vi "HT3_Open.vi"(8 "error in":errorcluster, 11 "File Path":path) -> (0 "error out":errorcluster, 1 "Num Records":i64, 2 "Header":T2, 3 "refnum out":refnum<file>, 4 "Stop After (ms)":i32, 5 "Stop Reason":enum16{"timeover", "manual", "overflow"}(ring), 7 "Image Header":T1)   [LabVIEW 2009]
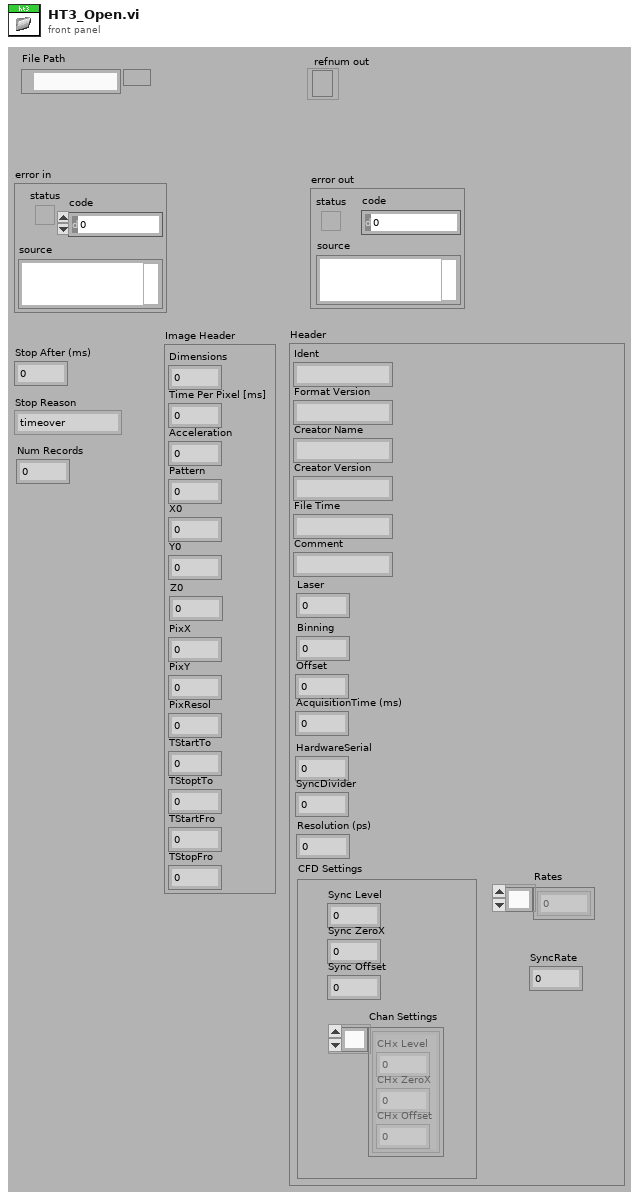
[diagram p1: front panel]
types:
  T1 = cluster{"Dimensions":i32, "Time Per Pixel [ms]":dbl, "Acceleration":i32, "Pattern":i32, "X0":sgl, "Y0":sgl, "Z0":dbl, "PixX":i32, "PixY":i32, "PixResol":sgl, "TStartTo":sgl, "TStoptTo":sgl, "TStartFro":sgl, "TStopFro":sgl}
  T2 = cluster{"Ident":string, "Format Version":string, "Creator Name":string, "Creator Version":string, "File Time":string, "Comment":string, "Laser":i32, "Binning":i32, "Offset":i32, "AcquisitionTime (ms)":i32, "HardwareSerial":i32, "SyncDivider":i32, "Resolution (ps)":dbl, "Rates":dbl[], "SyncRate":dbl, "CFD Settings":cluster{"Sync Level":i32, "Sync ZeroX":i32, "Sync Offset":i32, "Chan Settings":cluster{"CHx Level":i32, "CHx ZeroX":i32, "CHx Offset":i32}[]}}
  T3 = cluster{"Sync Level":i32, "Sync ZeroX":i32, "Sync Offset":i32, "Chan Settings":cluster{"CHx Level":i32, "CHx ZeroX":i32, "CHx Offset":i32}[]}
  T4 = cluster{"Ident":string, "Format Version":string, "Creator Name":string, "Creator Version":string, "File Time":string, "Comment":string, i32, "Binning":i32, "Offset":i32, "AcquisitionTime (ms)":i32, "HardwareSerial":i32, "SyncDivider":i32, "Resolution (ps)":dbl, i32[], "InpRate1":i32, "CFD Settings":cluster{"Sync Level":i32, "Sync ZeroX":i32, "Sync Offset":i32, "Chan Settings":cluster{"CHx Level":i32, "CHx ZeroX":i32, "CHx Offset":i32}[]}}
  T5 = enum16{"big-endian, network order", "native, host order", "little-endian"}
  T6 = enum16{"open", "replace", "create", "open or create", "replace or create", "replace or create with confirmation"}
  T7 = cluster{"Dimensions":i32, "Time Per Pixel [ms]":dbl, "Acceleration":i32, "Pattern":i32, "X0":sgl, "Y0":sgl, dbl, "PixX":i32, "PixY":i32, "PixResol":sgl, "TStartTo":sgl, "TStoptTo":sgl, "TStartFro":sgl, "TStopFro":sgl}
  T8 = cluster{"Strings[0]":string, "Strings[1]":string, "Strings[2]":string, "Strings[3]":string, "Strings[4]":string, "Strings[5]":string}
  T9 = cluster{"[0]":i32, "[1]":i32, "[2]":i32, "[3]":i32}
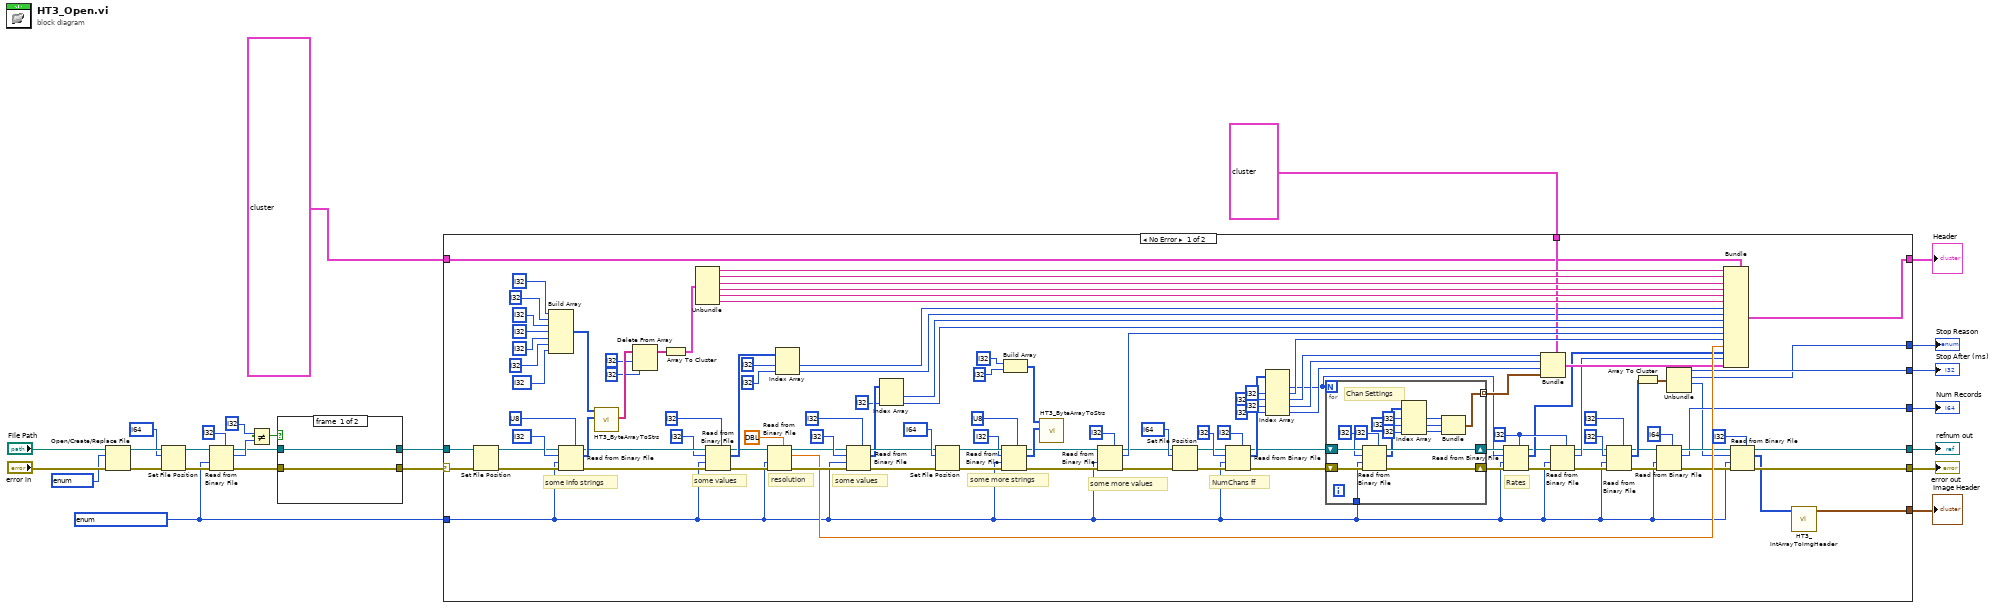
[diagram p0: block diagram]
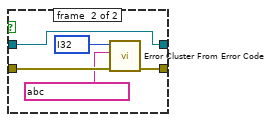
[diagram p2: hidden frame]
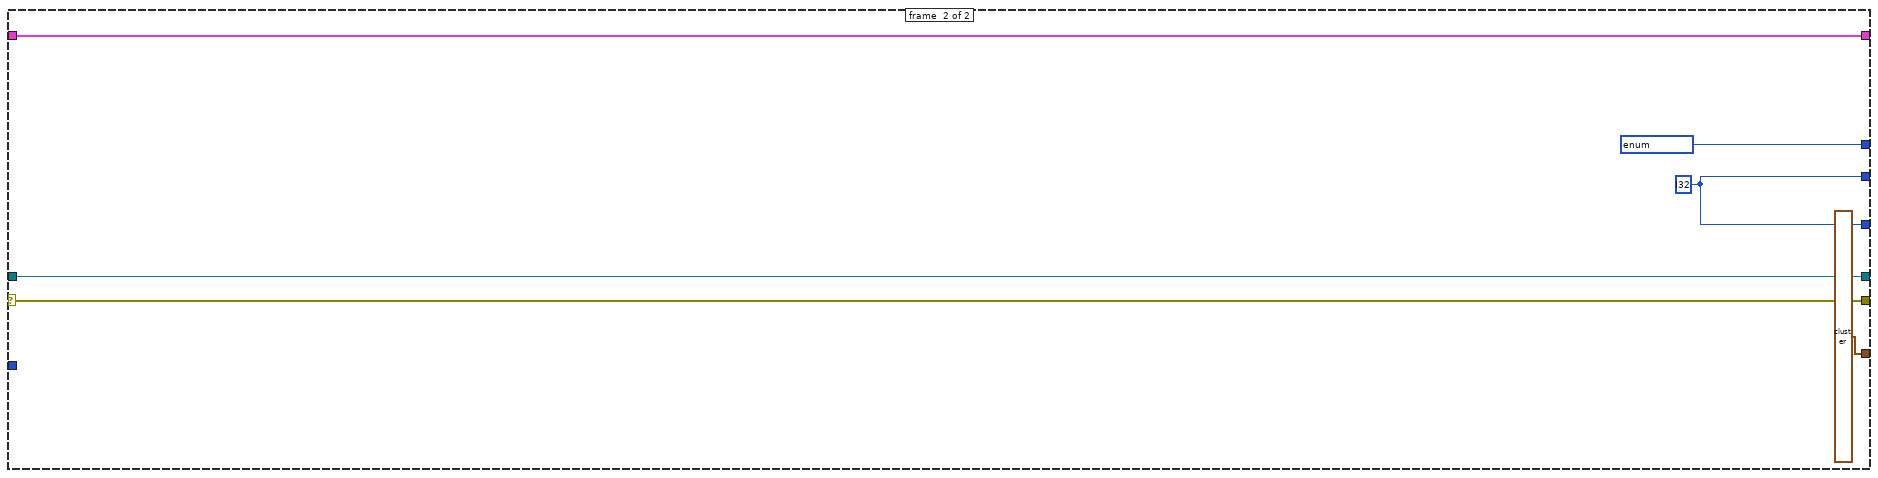
[diagram p3: hidden frame]
diagram:
  w12 = T5 ? ("byte order (0:big-endian, network order)")
  n1 = Open/Create/Replace File(file path (use dialog)="File Path", error in="error in", operation (0:open)=T6 ?) -> (refnum out=w15:refnum<file>, error out=w16:errorcluster)  [unwired: 4 out]
  n2 = Set File Position(offset (in bytes) (0)=i64 ?, refnum=w15, error in=w16) -> (refnum out=w11:refnum<file>, error out=w13:errorcluster)  [unwired: 1 out]
  n3 = Read from Binary File(5:i32 ?, 8:w13, 9:w12, 11:w11) -> (0:w6:errorcluster, 2:w9:i32, 3:w3:refnum<file>)  [unwired: 3 out]
  n4 = Not Equal?(x=i32 ?, y=w9) -> (x != y?=w7:bool)
  n5 = case shown="True" w7 {
    tunnel: w6 -> [w28 w33]
    tunnel: [w28 w32] -> w5
    tunnel: [w27 w29] -> w4
    tunnel: w3 -> [w27 w29]
    frame #0 {
    }
    frame #1 {
      n6 = call <vilib>:"Error Cluster From Error Code.vi"("error in (no error)"=w33, "error message (\"\")"=string ? ("error message (\"\")"), "error code (0)"=i32 ?) -> ("error out"=w32:errorcluster)  [unwired: 1 in, 5 out]
    }
  }
  n7 = case shown="No Error" w5 {
    selector: w5 -> [w130 w168]
    tunnel: [w97 w168] -> w23
    tunnel: [w96 w167] -> w22
    tunnel: w4 -> [w128 w167]
    tunnel: w12 -> [w47 _]
    tunnel: [w122 w164] -> w21
    tunnel: [w38 enum16{"timeover", "manual", "overflow"} ? ("Stop Reason")] -> w20
    tunnel: [w39 w165] -> w19
    tunnel: [w50 w165] -> w18
    tunnel: T4 ? ("Header") -> [w43 w164]
    tunnel: [w94 T7 ? ("Image Header")] -> w2
    tunnel: T3 ? ("CFD Settings") -> [w67 _]
    frame #0 {
      w48 = i32 ?
      # "Rates"
      # "NumChans ff"
      # "some values"
      # "resolution"
      # "some more values"
      # "some more strings"
      # "some values"
      # "some info strings"
      n8 = Set File Position(refnum=w128, error in=w130) -> (refnum out=w127:refnum<file>, error out=w129:errorcluster)  [unwired: 2 out]
      n9 = Build Array(i32 ? ("Length"), i32 ? ("Length"), i32 ? ("Length"), i32 ? ("Length"), i32 ? ("Length"), i32 ? ("Length"), i32 ? ("Length")) -> (w137:i32[])
      n10 = Read from Binary File(5:u8 ?, 8:w129, 9:w47, 10:i32 ? ("count (1)"), 11:w127) -> (0:w132:errorcluster, 2:w145:u8[], 3:w131:refnum<file>)  [unwired: 2 out]
      n11 = call "HT3_ByteArrayToStrs.vi"("Byte Array"=w145, "Lengths"=w137) -> ("Strings"=w136:string[])  [unwired: 9 out]
      n12 = Delete From Array(array=w136, length=i32 ?, index=i32 ?) -> (array with subset deleted=w133:string[])  [unwired: 1 out]
      n13 = Array To Cluster(array=w133) -> (cluster=w121:T8)
      n14 = Unbundle(w121) -> ("Strings[0]"=w120:string, "Strings[1]"=w119:string, "Strings[2]"=w118:string, "Strings[3]"=w117:string, "Strings[4]"=w116:string, "Strings[5]"=w115:string)
      n15 = Read from Binary File(5:i32 ?, 8:w132, 9:w47, 10:i32 ? ("count (1)"), 11:w131) -> (0:w92:errorcluster, 2:w124:i32[], 3:w91:refnum<file>)  [unwired: 2 out]
      n16 = Read from Binary File(5:dbl ? ("Resolution (ns)"), 8:w92, 9:w47, 11:w91) -> (0:w88:errorcluster, 2:w80:dbl, 3:w86:refnum<file>)  [unwired: 1 in, 2 out]
      n17 = Index Array(array=w124, index #1=i32 ? ("index"), index #2=i32 ?) -> (element #1=w34:i32, element #2=w35:i32)
      n18 = Read from Binary File(5:i32 ?, 8:w88, 9:w47, 10:i32 ? ("count (1)"), 11:w86) -> (0:w87:errorcluster, 2:w84:i32[], 3:w85:refnum<file>)  [unwired: 1 in, 1 out]
      n19 = Index Array(array=w84, index #2=i32 ? ("index")) -> (element #1=w82:i32, element #2=w81:i32)  [unwired: 1 in]
      n20 = Set File Position(offset (in bytes) (0)=i64 ?, refnum=w85, error in=w87) -> (refnum out=w112:refnum<file>, error out=w113:errorcluster)  [unwired: 1 out]
      n21 = Read from Binary File(5:u8 ?, 8:w113, 9:w47, 10:i32 ? ("count (1)"), 11:w112) -> (0:w105:errorcluster, 2:w109:u8[], 3:w104:refnum<file>)  [unwired: 2 out]
      n22 = Build Array(i32 ? ("Length"), i32 ? ("Length")) -> (w106:i32[])
      n23 = call "HT3_ByteArrayToStrs.vi"("Byte Array"=w109, "Lengths"=w106) -> ()  [unwired: 10 out]
      n24 = Read from Binary File(5:i32 ?, 8:w105, 9:w47, 11:w104) -> (0:w77:errorcluster, 2:w79:i32, 3:w76:refnum<file>)  [unwired: 1 in, 2 out]
      n25 = Set File Position(offset (in bytes) (0)=i64 ?, refnum=w76, error in=w77) -> (refnum out=w42:refnum<file>, error out=w74:errorcluster)  [unwired: 1 out]
      n26 = Read from Binary File(5:i32 ?, 8:w74, 9:w47, 10:i32 ? ("count (1)"), 11:w42) -> (0:w71:errorcluster, 2:w72:i32[], 3:w68:refnum<file>)  [unwired: 2 out]
      n27 = Index Array(array=w72, index #2=i32 ? ("index"), index #3=i32 ? ("index"), index #4=i32 ? ("index"), index #5=i32 ? ("index")) -> (element #1=w46:i32, element #2=w69:i32, element #3=w62:i32, element #4=w61:i32, element #5=w63:i32)  [unwired: 1 in]
      n28 = for {
        N: w46 -> [_]
        shift-right: [w161] -> w58
        shift-left: w71 -> [w162]
        tunnel: w47 -> [w160]
        shift-right: [w158] -> w56
        shift-left: w68 -> [w159]
        tunnel: [w148] -> w60 mode=indexing
        # "Chan Settings"
        n29 = Read from Binary File(5:i32 ?, 8:w162, 9:w160, 10:i32 ? ("count (1)"), 11:w159) -> (0:w161:errorcluster, 2:w155:i32[], 3:w158:refnum<file>)  [unwired: 1 in, 1 out]
        n30 = Index Array(array=w155, index #1=i32 ? ("index"), index #2=i32 ? ("index"), index #3=i32 ? ("index")) -> (element #1=w151:i32, element #2=w150:i32, element #3=w149:i32)
        n31 = Bundle(w151, w150, w149) -> (w148:cluster{i32, i32, i32})  [unwired: 1 in]
      }
      n32 = Read from Binary File(5:w48, 8:w58, 9:w47, 10:w46, 11:w56) -> (0:w57:errorcluster, 2:w45:i32[], 3:w41:refnum<file>)  [unwired: 2 out]
      n33 = Bundle(cluster=w67, "Sync Level"=w62, "Sync ZeroX"=w61, "Sync Offset"=w63, "Chan Settings"=w60) -> (w59:T3)
      n34 = Read from Binary File(5:w48, 8:w57, 9:w47, 11:w41) -> (0:w49:errorcluster, 2:w44:i32, 3:w40:refnum<file>)  [unwired: 2 in, 1 out]
      n35 = Read from Binary File(5:i32 ?, 8:w49, 9:w47, 10:i32 ? ("count (1)"), 11:w40) -> (0:w55:errorcluster, 2:w99:i32[], 3:w53:refnum<file>)  [unwired: 2 out]
      n36 = Array To Cluster(array=w99) -> (cluster=w100:T9)
      n37 = Read from Binary File(5:i64 ?, 8:w55, 9:w47, 11:w53) -> (0:w54:errorcluster, 2:w50:i64, 3:w52:refnum<file>)  [unwired: 1 in, 2 out]
      n38 = Unbundle(w100) -> ("[0]"=w39:i32, "[1]"=w38:i32, "[2]"=w37:i32)  [unwired: 1 out]
      n39 = Bundle(cluster=w43, "Ident"=w120, "Format Version"=w119, "Creator Name"=w118, "Creator Version"=w117, "File Time"=w116, "Comment"=w115, w34, "Binning"=w35, "Offset"=w82, "AcquisitionTime (ms)"=w81, "HardwareSerial"=w79, "SyncDivider"=w69, "Resolution (ps)"=w80, w45, "InpRate1"=w44, "CFD Settings"=w59) -> (w122:T4)
      n40 = Read from Binary File(5:i32 ?, 8:w54, 9:w47, 10:w37, 11:w52) -> (0:w97:errorcluster, 2:w95:i32[], 3:w96:refnum<file>)  [unwired: 2 out]
      n41 = call "HT3_IntArrayToImgHeader.vi"("Array"=w95) -> ("Image Header"=w94:T1)  [unwired: 10 out]
    }
    frame #1 {
      w165 = i32 ? ("Stop After (ms)")
    }
  }
  "refnum out" <- w22
  "error out" <- w23
  "Header" <- w21
  "Stop Reason" <- w20
  "Stop After (ms)" <- w19
  "Num Records" <- w18
  "Image Header" <- w2
